vi "Message for Extracting Info.vi"(1 "eHS Core Index":T1, 5 "Model Name":string, 7 "Minimum Ts":string, 9 "Number of Switchs":string, 11 "Error In":errorcluster) -> (4 "Message":string, 15 "Error Out":errorcluster)   [LabVIEW 2017]
uses:
  <vilib>/OPAL-RT/eHS Toolkit/eHS Matrix Generation/_Controls/eHS Core Index.ctl
  <vilib>/OPAL-RT/eHS Toolkit/eHS Matrix Generation/eHS Matrix Generation.lvlib
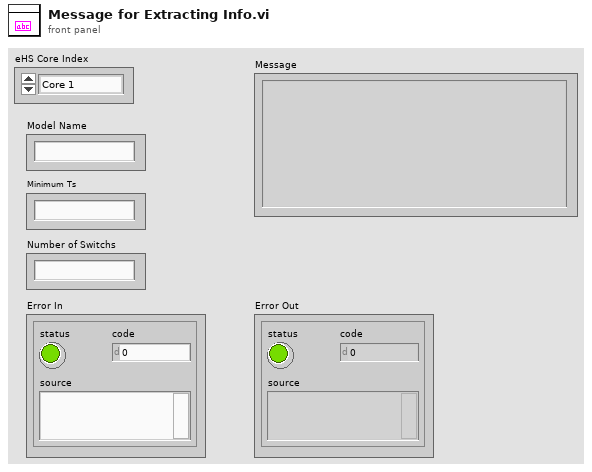
[diagram p1: front panel]
types:
  T1 = typedef "OPAL-RT eHS.lvlib/eHS Matrix Generation.lvlib/eHS Core Index.ctl" = enum16{"Core 1", "Core 2", "Core 3", "Core 4", "Core 5", "Core 6", "Core 7", "Core 8", "Core 9", "Core 10"}
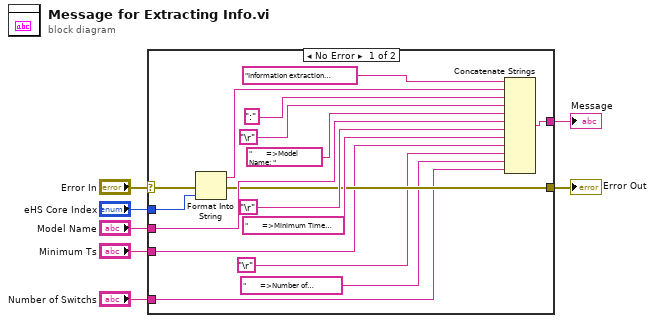
[diagram p0: block diagram]
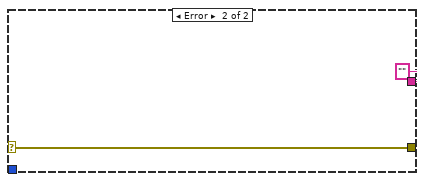
[diagram p2: hidden frame]
diagram:
  n1 = case shown="No Error" "Error In" {
    selector: "Error In" -> [w22 w25]
    tunnel: [w12 w25] -> w6
    tunnel: [w23 ""] -> w5
    tunnel: "eHS Core Index" -> [w21 _]
    tunnel: "Model Name" -> [w15 _]
    tunnel: "Minimum Ts" -> [w11 _]
    tunnel: "Number of Switchs" -> [w9 _]
    frame No Error {
      n2 = Format Into String(error in=w22, w21) -> (resulting string=w19:string, error out=w12:errorcluster)  [unwired: 2 in]
      n3 = Concatenate Strings("Information extraction complete for " ("string"), w19, ":" ("string"), "\r", "       =>Model Name: " ("string"), w15, "\r", "       =>Minimum Time Step:" ("string"), w11, "\r", "       =>Number of Switches:" ("string"), w9) -> (w23:string)
    }
    frame Error {
    }
  }
  "Error Out" <- w6
  "Message" <- w5
